vi "svm test.vi"() -> ()   [LabVIEW 2018]
doc: "Svm test: This example is a testing example of support vector machine, which uses a support vector machine model to classify or regress new data samples."
uses:
  vi.lib/VIRobotics/opencv_yiku/Mat/Mat_32F/Mat_32F.lvclass
  D:/Program Files/company/National Instruments/LabVIEW 2018/vi.lib/addons/VIRobotics/opencv_yiku/Mat/Mat/Mat.lvclass
  vi.lib/VIRobotics/opencv_yiku/Mat/Mat_32S/Mat_32S.lvclass
  vi.lib/VIRobotics/opencv_yiku/ml/SVM/setType.vi
  vi.lib/VIRobotics/opencv_yiku/ml/SVM/setKernel.vi
  vi.lib/VIRobotics/opencv_yiku/ml/SVM/setTermCriteria.vi
  vi.lib/VIRobotics/opencv_yiku/Mat/Create_Mat_32F.vi
  vi.lib/VIRobotics/opencv_yiku/Mat/Mat_32F/set_2d_data.vi
  vi.lib/VIRobotics/opencv_yiku/Mat/Create_Mat_32S.vi
  vi.lib/VIRobotics/opencv_yiku/ml/SVM/SVM_release.vi
  vi.lib/VIRobotics/opencv_yiku/ml/SVM/SVM.lvclass
  vi.lib/VIRobotics/opencv_yiku/opencv_yiku.lvlib
panel:
  out "Intensity Graph":sgl[][](graph)
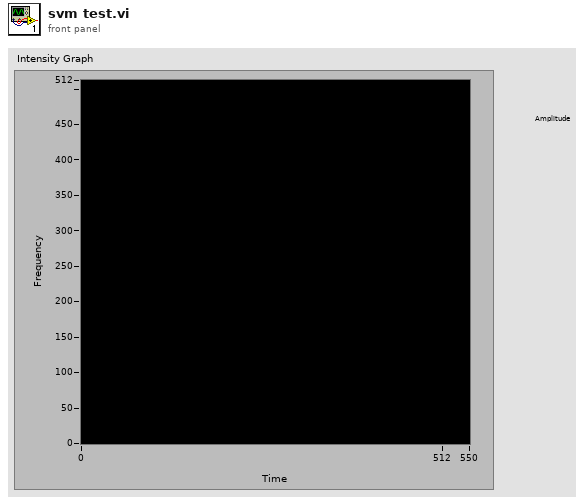
[diagram p1: front panel]
types:
  T1 = cluster{"type":i32, "maxCount":i32, "epsilon":dbl}
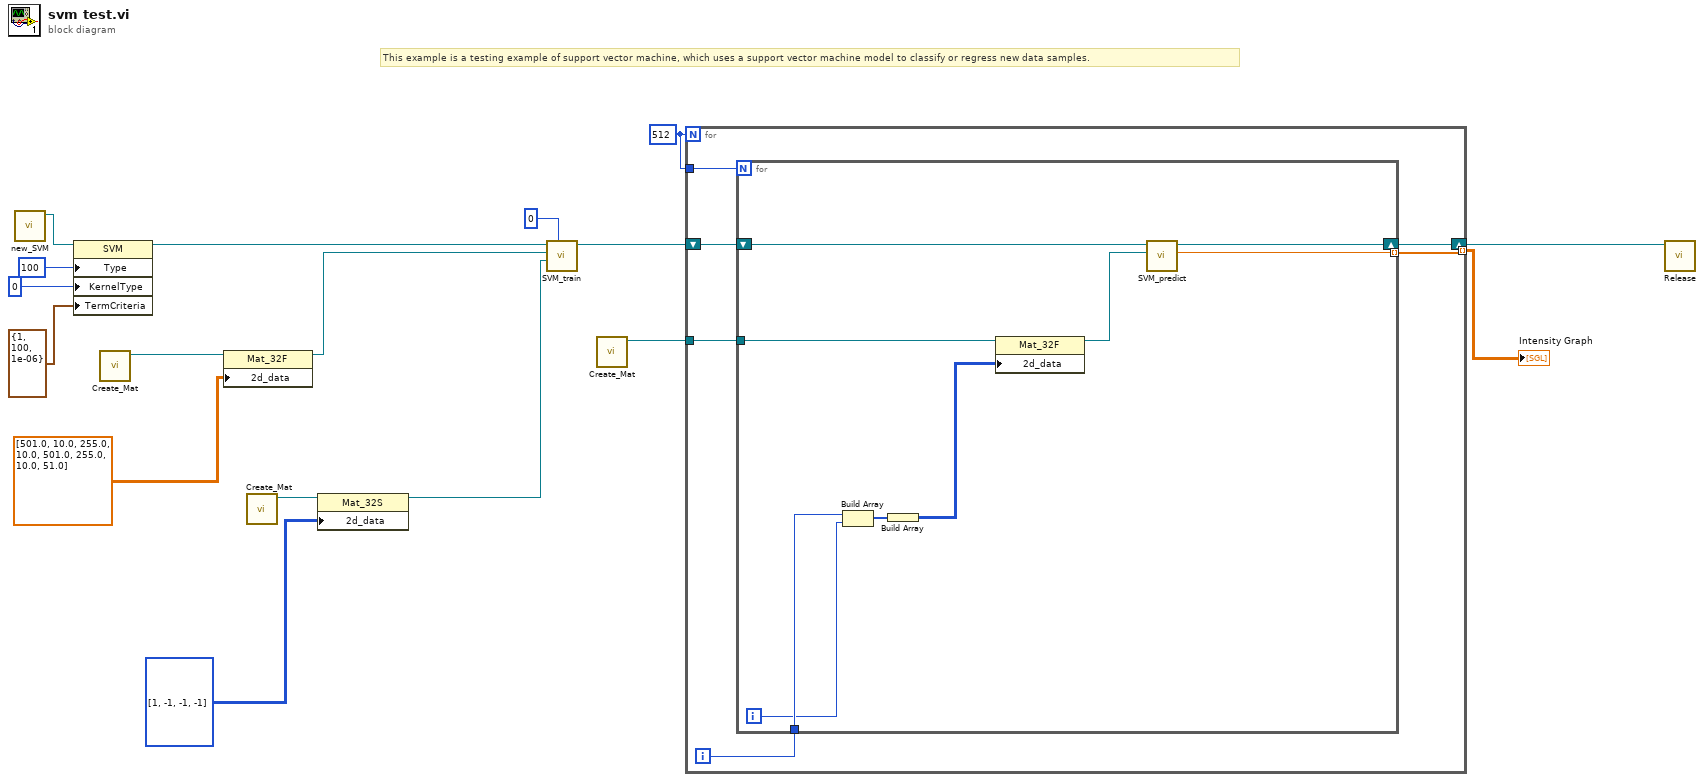
[diagram p0: block diagram]
diagram:
  w3 = 512
  # "This example is a testing example of support vector machine, which uses a support vector machine model to classify or regress new data samples."
  n1 = call "new_SVM.vi"() -> ("SVM out"=w14:refnum<class "SVM.lvclass">)  [unwired: 10 in, 1 out]
  n2 = property class="SVM"(reference=w14, "Type"=100, "KernelType"=0, "TermCriteria"=T1 {"type"=1, "maxCount"=100, "epsilon"=1e-06}) -> (reference out=w4:refnum<class "SVM.lvclass">)  [unwired: 1 in, 1 out]
  n3 = call-poly "Create_Mat.vi"() -> ("Mat_32F_out"=w13:refnum<class "Mat_32F.lvclass">)  [unwired: 10 in, 1 out]
  n4 = property class="Mat_32F"(reference=w13, "2d_data"=sgl[][] [[501.0, 10.0], [255.0, 10.0], [501.0, 255.0], [10.0, 51.0]]) -> (reference out=w9:refnum<class "Mat_32F.lvclass">)  [unwired: 1 in, 1 out]
  n5 = call-poly "Create_Mat.vi"() -> ("Mat_32S_out"=w11:refnum<class "Mat_32S.lvclass">)  [unwired: 10 in, 1 out]
  n6 = property class="Mat_32S"(reference=w11, "2d_data"=i32[][] [[1], [-1], [-1], [-1]]) -> (reference out=w8:refnum<class "Mat_32S.lvclass">)  [unwired: 1 in, 1 out]
  n7 = call "SVM_train.vi"("layout"=0 ("type"), "label"=w8, "data"=w9, "SVM in"=w4) -> ("SVM out"=w6:refnum<class "SVM.lvclass">)  [unwired: 6 in, 1 out]
  n8 = call-poly "Create_Mat.vi"() -> ("Mat_32F_out"=w5:refnum<class "Mat_32F.lvclass">)  [unwired: 10 in, 1 out]
  n9 = for {
    N: w3 -> [_]
    tunnel: w5 -> [w22]
    tunnel: [w20] -> w2 mode=indexing
    tunnel: w3 -> [w19]
    shift-right: [w18] -> w1
    shift-left: w6 -> [w23]
    i -> [w21]
    n10 = for {
      N: w19 -> [_]
      tunnel: w22 -> [w31]
      tunnel: w21 -> [w29]
      tunnel: [w25] -> w20 mode=indexing
      shift-right: [w24] -> w18
      shift-left: w23 -> [w32]
      i -> [w28]
      n11 = Build Array(w29, w28) -> (w27:i32[])
      n12 = Build Array(w27) -> (w26:i32[][])
      n13 = property class="Mat_32F"(reference=w31, "2d_data"=w26) -> (reference out=w30:refnum<class "Mat_32F.lvclass">)  [unwired: 1 in, 1 out]
      n14 = call "SVM_predict.vi"("data"=w30, "SVM in"=w32) -> ("predict"=w25:sgl, "SVM out"=w24:refnum<class "SVM.lvclass">)  [unwired: 7 in, 1 out]
    }
  }
  "Intensity Graph" <- w2
  n15 = call-poly "Release.vi"("SVM in"=w1) -> ()  [unwired: 9 in, 2 out]
